vi "LabVIEW to Python code.vi"(8 "error in":errorcluster, 9 "Defines":string[](array[string]), 10 "Includes":string[](array[string]), 11 "vi path":path) -> (0 "error out":errorcluster, 3 "transcripted code":string)   [LabVIEW 2014]
panel:
  out "wires with breakpoints":string[](array[string])
  # "Use Arduino.h just for arduino\nNO for ESP8266!"
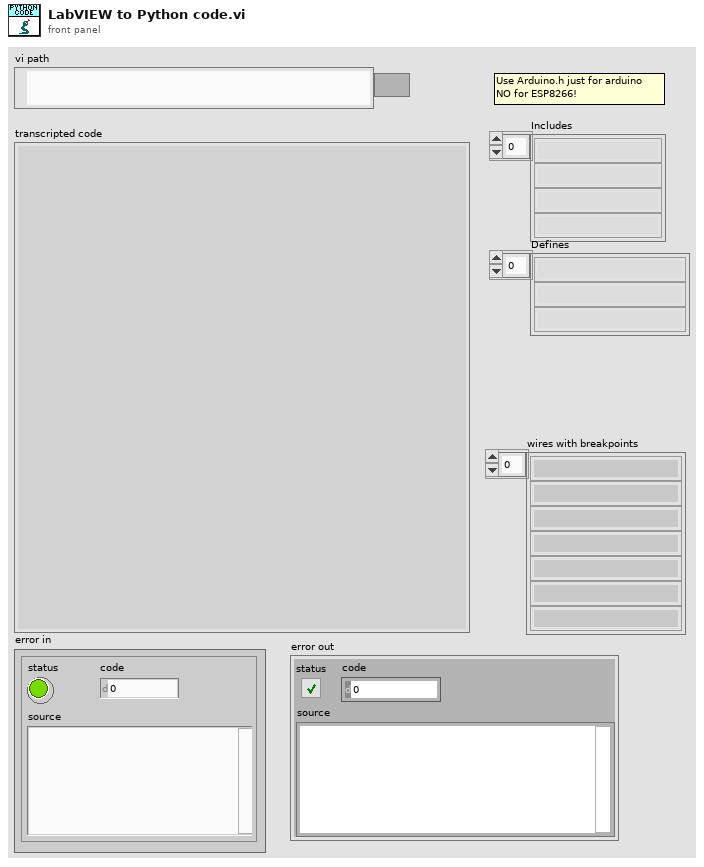
[diagram p1: front panel]
types:
  T1 = typedef "LabVIEW Universal Transcriptor Cluster.ctl" = cluster{"Defines":string[], "Includes":string[], "C code":string, "temp":string[], "temp 2":string[], "wires with breakpoints":string[]}
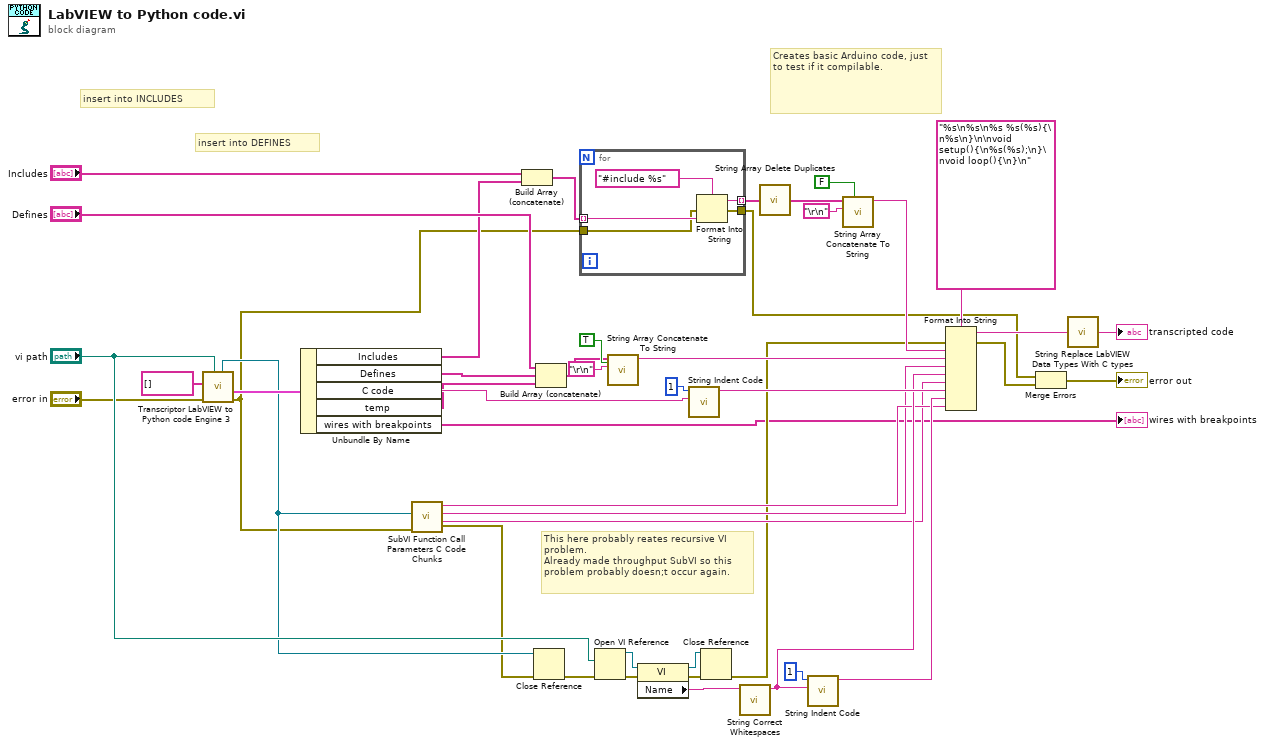
[diagram p0: block diagram]
diagram:
  # "This here probably reates recursive VI problem.\nAlready made throughput SubVI so this problem probably doesn;t occur again."
  # "insert into INCLUDES"
  # "insert into DEFINES"
  # "Creates basic Arduino code, just to test if it compilable."
  n1 = call "Transcriptor LabVIEW to Python code Engine 3.vi"("VI path"="vi path", "Error In"="error in", "List Reentrant VIs"=string[] []) -> ("error out"=w4:errorcluster, "output cluster"=w45:T1, "VI ref."=w12:refnum<vi>)  [unwired: 4 in, 2 out]
  n2 = Unbundle By Name(w45) -> ("Includes"=w23:string[], "Defines"=w26:string[], "C code"=w34:string, "temp"=w14:string[], "wires with breakpoints"=→"wires with breakpoints":string[])
  n3 = call "SubVI Function Call Parameters C Code Chunks.vi"("Error In"=w4, "VI Reference"=w12) -> ("SubVI func. declaration"=w18:string, "return datatype"=w19:string, "SubVI func. call in code"=w20:string, "Error Out"=w11:errorcluster)  [unwired: 4 in, 2 out]
  n4 = Build Array (concatenate)("Includes", w23) -> (w22:string[])
  n5 = Close Reference(reference=w12, error in (no error)=w11) -> (error out=w13:errorcluster)
  n6 = Build Array (concatenate)("Defines", w26, w14) -> (w25:string[])
  n7 = for {
    tunnel: w22 -> [w49] mode=indexing
    tunnel: [w48] -> w10 mode=indexing
    tunnel: w4 -> [w47]
    tunnel: [w46] -> w5
    n8 = Format Into String(format string="#include %s", error in=w47, w49) -> (resulting string=w48:string, error out=w46:errorcluster)  [unwired: 1 in]
  }
  n9 = Open VI Reference(vi path="vi path", error in (no error)=w13) -> (vi reference=w16:refnum<vi>, error out=w37:errorcluster)  [unwired: 4 in]
  n10 = call "String Array Concatenate To String.vi"("insert last delimiter?"=TRUE, "Delimiter char"="\r\n", "Array String In"=w25) -> ("String"=w42:string)  [unwired: 8 in]
  n11 = property class="VI"(reference=w16, error in=w37) -> (reference out=w17:refnum<vi>, error out=w35:errorcluster, "Name"=w36:string)
  n12 = call "String Indent Code.vi"("complete code"=w34, "actual nested level"=1) -> ("indented code"=w33:string)  [unwired: 9 in]
  n13 = Close Reference(reference=w17, error in (no error)=w35) -> (error out=w8:errorcluster)
  n14 = call "String Correct Whitespaces.vi"("String in"=w36) -> ("String out"=w30:string)  [unwired: 10 in]
  n15 = call "String Array Delete Duplicates.vi"("Array"=w10) -> ("Output array"=w9:string[])
  n16 = call "String Indent Code.vi"("complete code"=w30, "actual nested level"=1) -> ("indented code"=w29:string)  [unwired: 9 in]
  n17 = call "String Array Concatenate To String.vi"("insert last delimiter?"=FALSE, "Delimiter char"="\r\n", "Array String In"=w9) -> ("String"=w38:string)  [unwired: 8 in]
  n18 = Format Into String(format string="%s\n%s\n%s %s(%s){\n%s\n}\n\nvoid setup(){\n%s(%s);\n}\nvoid loop(){\n}\n", error in=w8, w38, w42, w19, w30, w18, w33, w29, w20) -> (resulting string=w28:string, error out=w6:errorcluster)  [unwired: 1 in]
  n19 = Merge Errors(w5, w6) -> (→"error out":errorcluster)
  n20 = call "String Replace LabVIEW Data Types With C types.vi"("C code"=w28) -> ("C code, replaced datatypes"=→"transcripted code":string)
